vi "Protype.vi"() -> ()   [LabVIEW 2020]
panel:
  out "Common":string
  out "Not in Reference":string[](array[string])
  out "Not in Target":string[](array[string])
  out "Not in Ref":T1(array[cluster])
  in  "Reference":string
  in  "Target":string
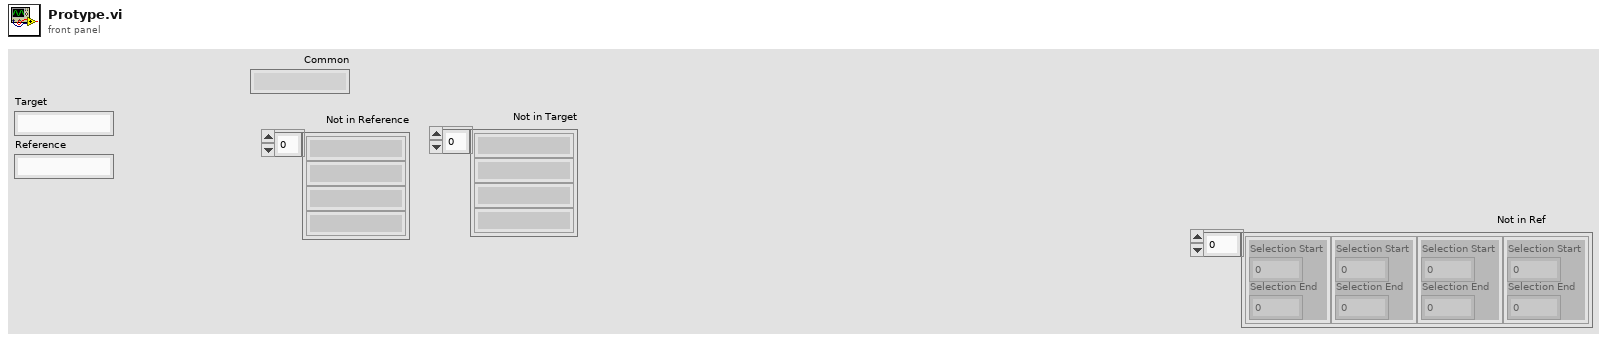
[diagram p1: front panel]
types:
  T1 = cluster{"Selection Start":u32, "Selection End":u32}[]
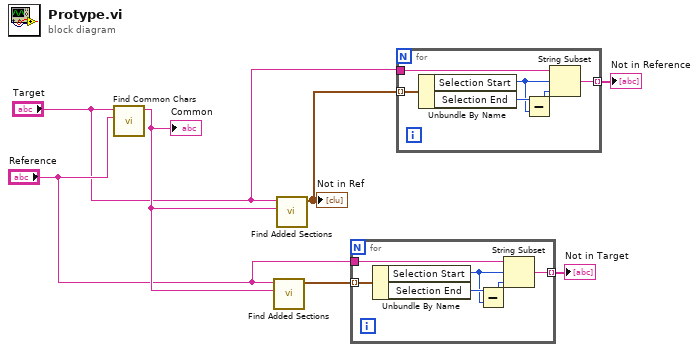
[diagram p0: block diagram]
diagram:
  n1 = call "Find Common Chars.vi"("Reference"="Reference", "Target"="Target") -> ("Common"=w7:string)  [unwired: 9 in]
  "Common" <- w7
  n2 = call "Find Added Sections.vi"("Reference"=w7, "Target"="Reference") -> ("Sections in Target"=w5:T1)  [unwired: 9 in]
  n3 = call "Find Added Sections.vi"("Reference"=w7, "Target"="Target") -> ("Sections in Target"=w2:T1)  [unwired: 9 in]
  "Not in Ref" <- w2
  n4 = for {
    tunnel: "Reference" -> [w13]
    tunnel: w5 -> [w12] mode=indexing
    tunnel: [w8] -> w4 mode=indexing
    n5 = Unbundle By Name(w12) -> ("Selection Start"=w10:u32, "Selection End"=w11:u32)
    n6 = Subtract(x=w11, y=w10) -> (x-y=w9:u32)
    n7 = String Subset(string=w13, offset (0)=w10, length (rest)=w9) -> (substring=w8:string)
  }
  "Not in Target" <- w4
  n8 = for {
    tunnel: "Target" -> [w19]
    tunnel: w2 -> [w18] mode=indexing
    tunnel: [w14] -> w3 mode=indexing
    n9 = Unbundle By Name(w18) -> ("Selection Start"=w16:u32, "Selection End"=w17:u32)
    n10 = Subtract(x=w17, y=w16) -> (x-y=w15:u32)
    n11 = String Subset(string=w19, offset (0)=w16, length (rest)=w15) -> (substring=w14:string)
  }
  "Not in Reference" <- w3
